vi "GetLaserData.vi"(11 "Path to Insight laser calibration folder":path=path "C:/Users/User/Documents/Insight_1310") -> (0 "DVV":dbl[](array[numeric]), 1 "DVV array size":i32, 3 "Laser parameters":T1)   [LabVIEW 2016]
uses:
  CTL/Laser_Parameters.ctl
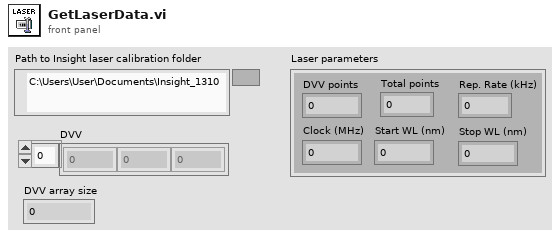
[diagram p1: front panel]
types:
  T1 = typedef "Laser_Parameters.ctl" = cluster{"DVV points":dbl, "Total points":dbl, "Rep. Rate (kHz)":dbl, "Clock (MHz)":dbl, "Start WL (nm) ":dbl, "Stop WL (nm)":dbl}
  T2 = cluster{"array type (2D Dbl)[0]":dbl, "array type (2D Dbl)[1]":dbl, "array type (2D Dbl)[2]":dbl, "array type (2D Dbl)[3]":dbl, "array type (2D Dbl)[4]":dbl, "array type (2D Dbl)[5]":dbl, "array type (2D Dbl)[6]":dbl, "array type (2D Dbl)[7]":dbl, "array type (2D Dbl)[8]":dbl, "array type (2D Dbl)[9]":dbl, "array type (2D Dbl)[10]":dbl, "array type (2D Dbl)[11]":dbl}
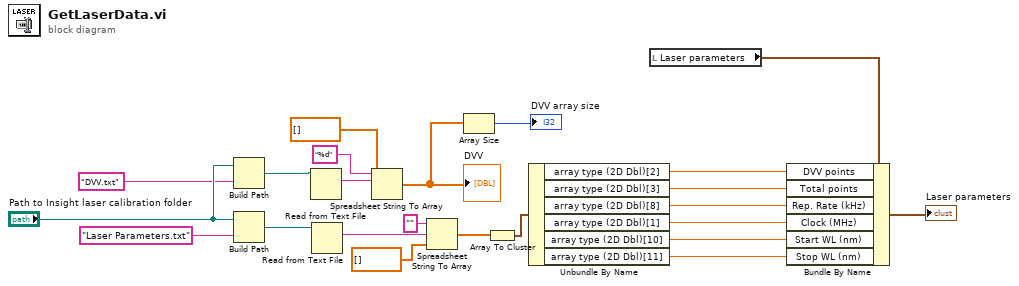
[diagram p0: block diagram]
diagram:
  n1 = Build Path(base path="Path to Insight laser calibration folder", name or relative path="DVV.txt") -> (appended path=w19:path)
  n2 = Build Path(base path="Path to Insight laser calibration folder", name or relative path="Laser Parameters.txt") -> (appended path=w22:path)
  n3 = Read from Text File(file (use dialog)=w19) -> (text=w18:string)  [unwired: 3 in, 3 out]
  n4 = Read from Text File(file (use dialog)=w22) -> (text=w16:string)  [unwired: 3 in, 3 out]
  n5 = Spreadsheet String To Array(format string="%d", spreadsheet string=w18, array type (2D Dbl)=dbl[] []) -> (array=w3:dbl[])  [unwired: 1 in]
  "DVV" <- w3
  n6 = Spreadsheet String To Array(format string="", spreadsheet string=w16, array type (2D Dbl)=dbl[] []) -> (array=w10:dbl[])  [unwired: 1 in]
  n7 = Array Size(array=w3) -> (size(s)=→"DVV array size":i32)
  n8 = Array To Cluster(array=w10) -> (cluster=w9:T2)
  n9 = Unbundle By Name(w9) -> ("array type (2D Dbl)[2]"=w2:dbl, "array type (2D Dbl)[3]"=w8:dbl, "array type (2D Dbl)[8]"=w7:dbl, "array type (2D Dbl)[1]"=w6:dbl, "array type (2D Dbl)[10]"=w5:dbl, "array type (2D Dbl)[11]"=w4:dbl)
  n10 = local read "Laser parameters"() -> (w14:T1)
  n11 = Bundle By Name(cluster=w14, "DVV points"=w2, "Total points"=w8, "Rep. Rate (kHz)"=w7, "Clock (MHz)"=w6, "Start WL (nm)"=w5, "Stop WL (nm)"=w4) -> (→"Laser parameters":T1)
